vi "Update Time Remaining Indicator.vi"(8 "error in (no error)":errorcluster, 10 "Time Remaining":dbl, 11 "Simulated Wash Display Console in":refnum<class "Simulated Wash Display Console.lvclass">) -> (0 "error out":errorcluster, 3 "Simulated Wash Display Console out":refnum<class "Simulated Wash Display Console.lvclass">)   [LabVIEW 2012, in "Simulated Wash Display Console.lvlib" / "Simulated Wash Display Console.lvclass"]
uses:
  Simulated Wash Display Console.lvclass
  Wash Display Console API/Wash Display Console API/Wash Display Console API.lvclass
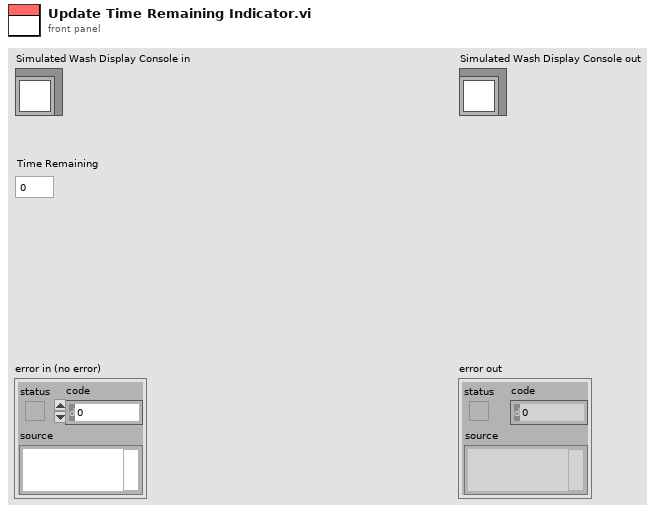
[diagram p1: front panel]
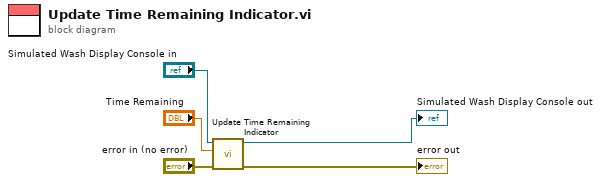
[diagram p0: block diagram]
diagram:
  n1 = call-parent "Update Time Remaining Indicator.vi"("error in (no error)"="error in (no error)", "Time Remaining"="Time Remaining", "Wash Display Console API in"="Simulated Wash Display Console in") -> ("error out"=→"error out":errorcluster, "Wash Display Console API out"=→"Simulated Wash Display Console out":refnum<class "Simulated Wash Display Console.lvclass">)  [unwired: 7 in]
